vi "complex multiply by fxp.vi"(9 "data in":u32, 10 "input valid":bool, 11 "Data A":fxp<+,16,0>) -> (1 "data valid":bool, 2 "Q":fxp<+/-,19,16>, 3 "I":fxp<+/-,19,16>)   [LabVIEW 2021]
uses:
  <vilib>/rvi/FXPMathLib/FxpMul/XNode/nifxpmath_Multiplier.xnode
  <vilib>/rvi/FXPMathLib/sim/FxpSim.dll
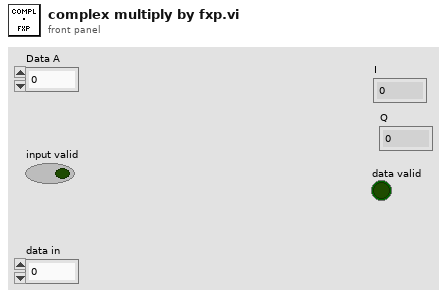
[diagram p1: front panel]
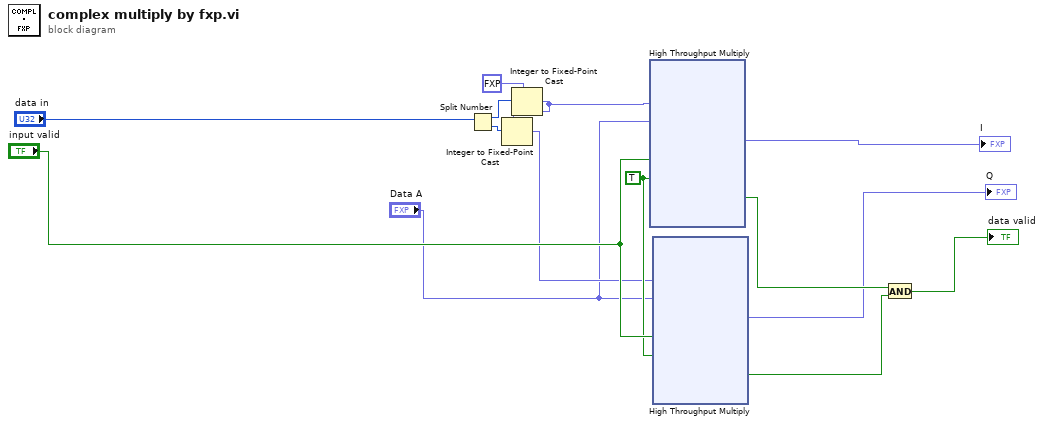
[diagram p0: block diagram]
diagram:
  w13 = TRUE ("ready for output (T)")
  n1 = Split Number(x="data in") -> (hi(x)=w7:u16, lo(x)=w6:u16)
  n2 = Integer to Fixed-Point Cast(fixed-point type=fxp<+/-,16,16> 0.0, integer=w7) -> (fixed-point=w11:fxp<+/-,16,16>)
  n3 = Integer to Fixed-Point Cast(fixed-point type=w11, integer=w6) -> (fixed-point=w12:fxp<+/-,16,16>)
  n4 = xnode "High Throughput Multiply"("x"=w11, "y"="Data A", "input valid"="input valid", "ready for output (T)"=w13) -> ("x*y"=→"I":fxp<+/-,19,16>, "output valid"=w5:bool)  [unwired: 1 out]
  n5 = xnode "High Throughput Multiply"("x"=w12, "y"="Data A", "input valid"="input valid", "ready for output (T)"=w13) -> ("x*y"=→"Q":fxp<+/-,19,16>, "output valid"=w4:bool)  [unwired: 1 out]
  n6 = And(x=w5, y=w4) -> (x .and. y?=→"data valid":bool)
